vi "Depth.vi"(10 "Area 1 - Area 2":dbl) -> (2 "In Range?":bool)   [LabVIEW 2014]
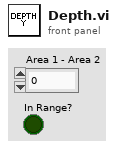
[diagram p1: front panel]
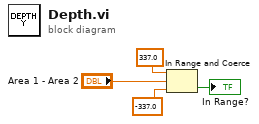
[diagram p0: block diagram]
diagram:
  n1 = In Range and Coerce(upper limit=337.0, x="Area 1 - Area 2", lower limit=-337.0) -> (In Range?=→"In Range?":bool)  [unwired: 1 out]
